vi "UnReserve.vi"(8 "error in (no error)":errorcluster, 9 "Job Results":T2 {"Status" items=["Service Error"=504, "Abort"=503, "Fail"=500, "Pass"=200]}, 11 "Executor":refnum<class "Executor.lvclass">) -> (0 "error out":errorcluster, 1 "Safe Shutdown?":bool, 2 "Executor States":T1[](array[typedef]), 3 "Executor":refnum<class "Executor.lvclass">)   [LabVIEW 2014, in "Executor.lvclass"]
doc: "This VI sets the Status to False and Sends the result to the job queue. The web Service Method is waiting indefinately for the Job Result"
uses:
  Executor.lvclass
  Controls/Job Results - STYP.ctl
  Controls/Executor Status - STYP.ctl
  Executor.lvclass/Executor.ctl
  Controls/Executor Data - STYP.ctl
  <vilib>/ActorFramework/Message Enqueuer/Message Enqueuer.lvclass
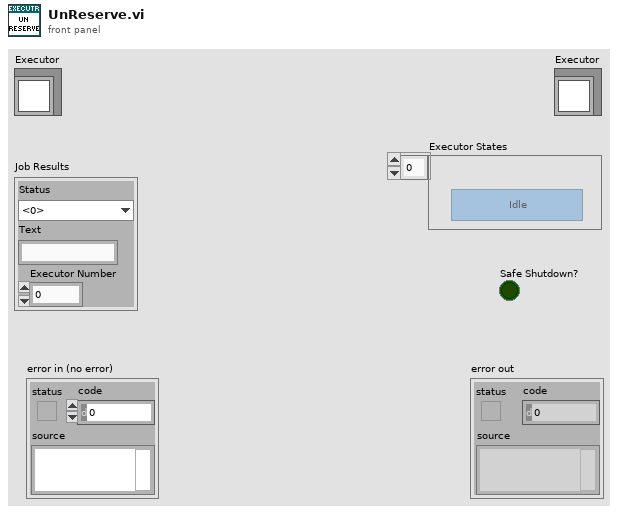
[diagram p1: front panel]
types:
  T1 = typedef "Executor Status - STYP.ctl" = cluster{"Executor Name":string, "Status":bool}
  T2 = typedef "Job Results - STYP.ctl" = cluster{"Status":u16, "Text":string, "Executor Number":i32}
  T3 = typedef "Executor Data - STYP.ctl" = cluster{"Status":T1, "Result Queue":refnum<queue>, "Actor Enquerer":refnum<class "Message Enqueuer.lvclass">}
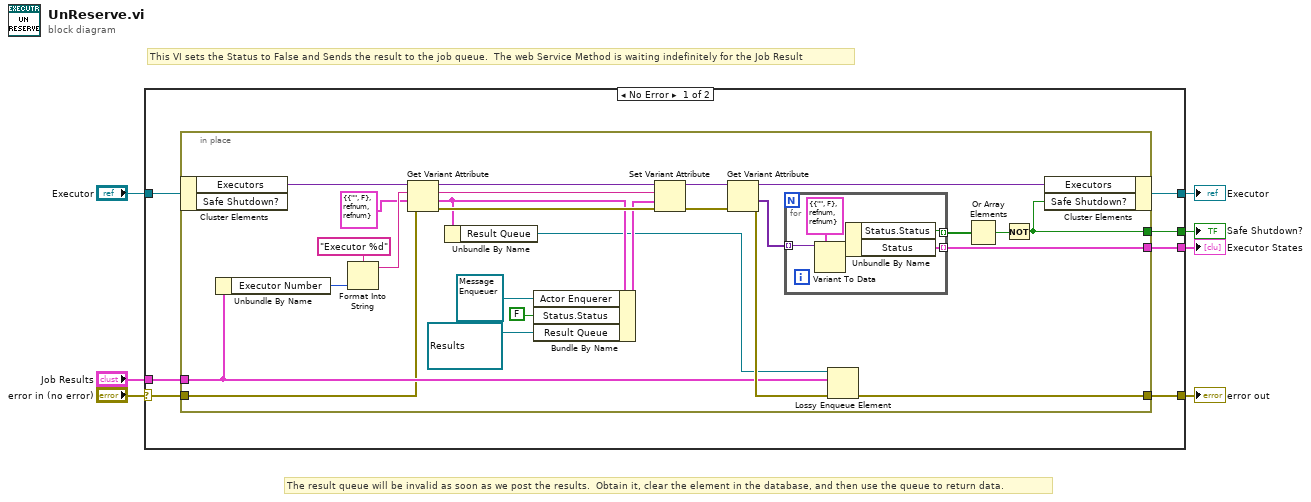
[diagram p0: block diagram]
diagram:
  # "The result queue will be invalid as soon as we post the results.  Obtain it, clear the element in the database, and then use the queue to return data."
  # "This VI sets the Status to False and Sends the result to the job queue.  The web Service Method is waiting indefinitely for the Job Result"
  n1 = case shown="No Error" "error in (no error)" {
    selector: "error in (no error)" -> [w9 w46]
    tunnel: [w13 w46] -> w6
    tunnel: [w11 w45] -> w4
    tunnel: "Executor" -> [w12 w45]
    tunnel: "Job Results" -> [w14 _]
    tunnel: [w10 _] -> w2
    tunnel: [w8 _] -> w1
    frame No Error {
      n2 = in-place {
        in-place-border: w14 -> [w24]
        in-place-border: [w27] -> w13
        in-place-border: [w20] -> w10
        in-place-border: w9 -> [w19]
        in-place-border: [w15] -> w8
        n3 = in-place-cluster #1(w12) -> ("Executors"=w39:variant)  [unwired: 1 out]
        n4 = Unbundle By Name(w24) -> ("Executor Number"=w23:i32)
        n5 = Format Into String(format string="Executor %d", w23) -> (resulting string=w37:string)  [unwired: 2 in, 1 out]
        n6 = Get Variant Attribute(Variant=w39, name=w37, default value (empty Variant)=T3 {"Status"={"Executor Name"="", "Status"=FALSE}, "Result Queue"=refnum, "Actor Enquerer"=refnum} ("Executor Data"), error in=w19) -> (duplicate Variant=w36:variant, value=w25:T3, error out=w33:errorcluster)  [unwired: 1 out]
        n7 = Unbundle By Name(w25) -> ("Result Queue"=w18:refnum<queue>)
        n8 = Bundle By Name(cluster=w25, "Actor Enquerer"=refnum<class "Message Enqueuer.lvclass"> refnum, "Status.Status"=FALSE ("Status"), "Result Queue"=refnum<queue> refnum) -> (w29:T3)
        n9 = Set Variant Attribute(Variant=w36, name=w37, value=w29, error in=w33) -> (Variant out=w35:variant, error out=w32:errorcluster)  [unwired: 1 out]
        n10 = Get Variant Attribute(Variant=w35, error in=w32) -> (duplicate Variant=w34:variant, values=w31:variant[], error out=w28:errorcluster)  [unwired: 2 in, 1 out]
        n11 = for {
          tunnel: w31 -> [w44] mode=indexing
          tunnel: [w41] -> w20 mode=indexing
          tunnel: [w40] -> w22 mode=indexing
          n12 = Variant To Data(type=T3 {"Status"={"Executor Name"="", "Status"=FALSE}, "Result Queue"=refnum, "Actor Enquerer"=refnum} ("Executor Data"), Variant=w44) -> (data=w42:T3)  [unwired: 1 in, 1 out]
          n13 = Unbundle By Name(w42) -> ("Status.Status"=w40:bool, "Status"=w41:T1)
        }
        n14 = Lossy Enqueue Element(queue=w18, element=w24, error in (no error)=w28) -> (error out=w27:errorcluster)  [unwired: 3 out]
        n15 = Or Array Elements(Boolean array=w22) -> (logical OR=w21:bool)
        n16 = Not(x=w21) -> (.not. x?=w15:bool)
        n17 = in-place-cluster #1("Executors"=w34, "Safe Shutdown?"=w15) -> (w11:refnum<class "Executor.lvclass">)
      }
    }
    frame Error {
    }
  }
  "error out" <- w6
  "Executor" <- w4
  "Executor States" <- w2
  "Safe Shutdown?" <- w1
